vi "Read Data.vi"(8 "error in (no error)":errorcluster, 11 "Alicat in":refnum<class "Alicat.lvclass">) -> (0 "error out":errorcluster, 2 "Data":refnum<class "Data.lvclass">, 3 "Alicat out":refnum<class "Alicat.lvclass">)   [LabVIEW 2015, in "Alicat.lvlib" / "Alicat.lvclass"]
uses:
  Alicat.lvclass
  Reusable/Data/Data.lvclass
  Alicat.lvclass/Alicat.ctl
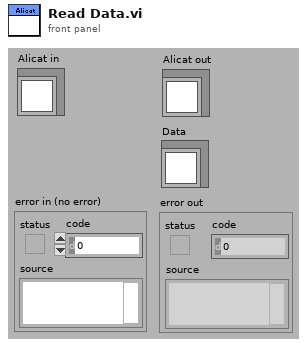
[diagram p1: front panel]
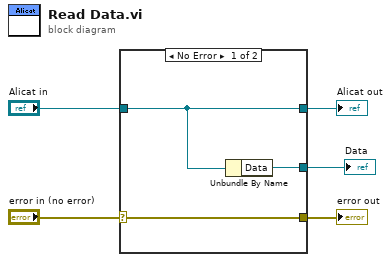
[diagram p0: block diagram]
diagram:
  n1 = case shown="No Error" "error in (no error)" {
    selector: "error in (no error)" -> [w8 w10]
    tunnel: [w8 w10] -> w4
    tunnel: [w7 w9] -> w2
    tunnel: "Alicat in" -> [w7 w9]
    tunnel: [w6 _] -> w1
    frame No Error {
      n2 = Unbundle By Name(w7) -> ("Data"=w6:refnum<class "Data.lvclass">)
    }
    frame Error {
    }
  }
  "error out" <- w4
  "Alicat out" <- w2
  "Data" <- w1
